vi "q-PCR report.vi"() -> ()   [LabVIEW 2017]
uses:
  <vilib>/addons/_office/excel.llb/Excel Get Data ([str]).vi
  <vilib>/Utility/NIReport.llb/Append Text Table to Report (wrap).vi
  <vilib>/Utility/NIReport.llb/NI_report.lvclass
  <vilib>/Utility/NIReport.llb/Excel/NI_Excel.lvclass
  <vilib>/addons/_office/NI_ReportGenerationToolkit.lvlib
panel:
  out "q-PCR Result":picture[][](array[picture])
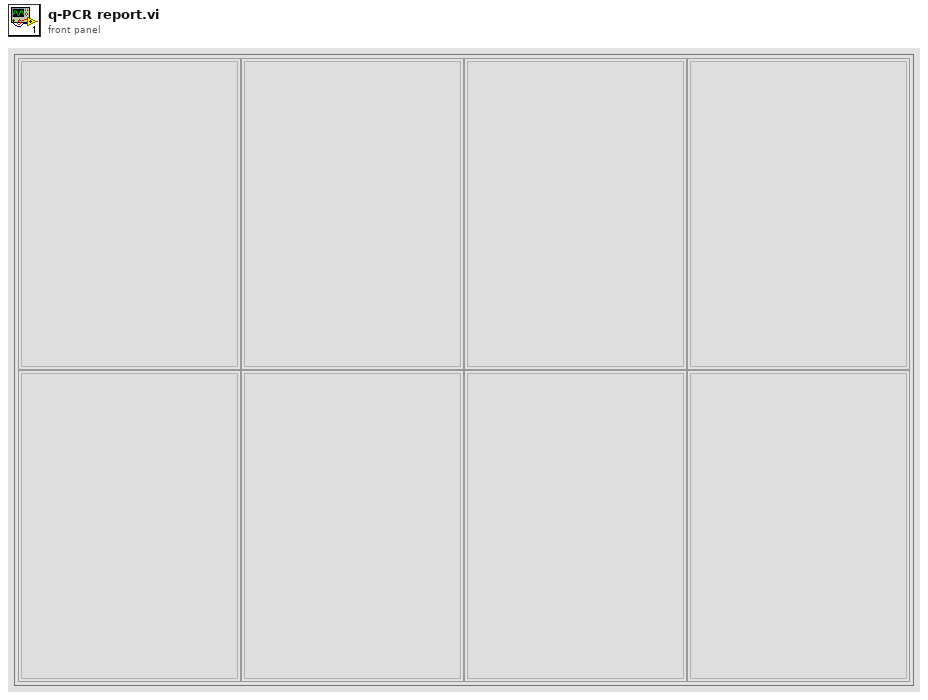
[diagram p1: front panel]
types:
  T1 = enum16{"Load File", "Plate Config", "Main Processing", "Report generation"}
  T2 = enum16{"maximized", "minimized", "normal", "no change"}
  T3 = enum16{"Standard Report", "HTML", "Word", "Excel"}
  T4 = cluster{"Group #":dbl, "Biological replicate":dbl, "Technical replicate":dbl}
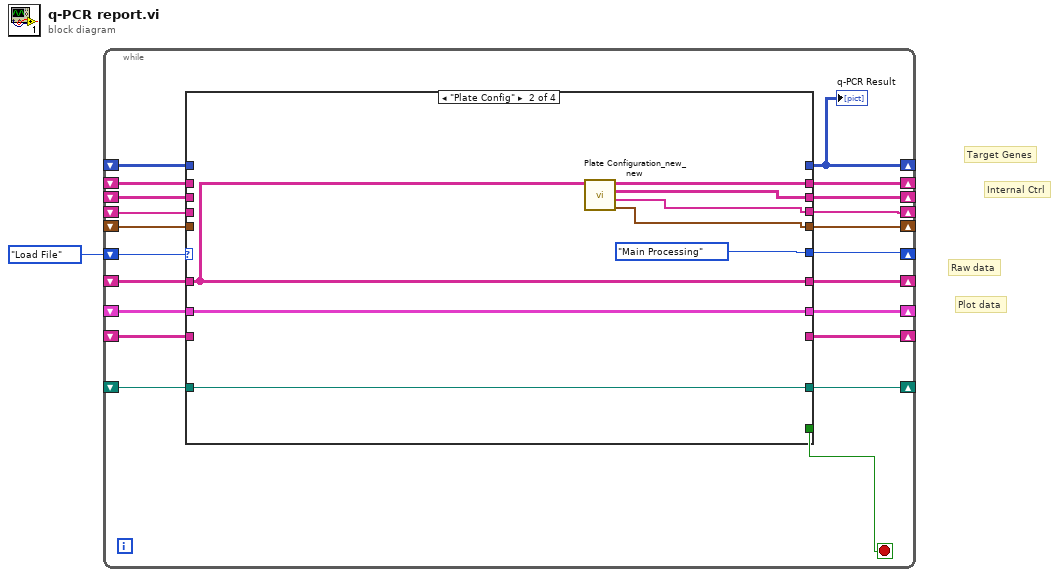
[diagram p0: block diagram]
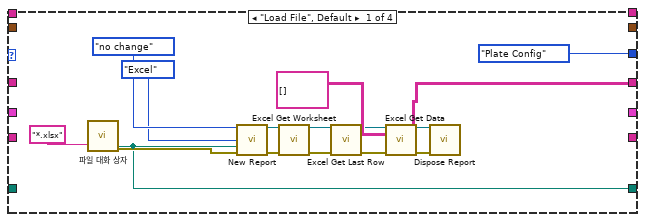
[diagram p2: hidden frame]
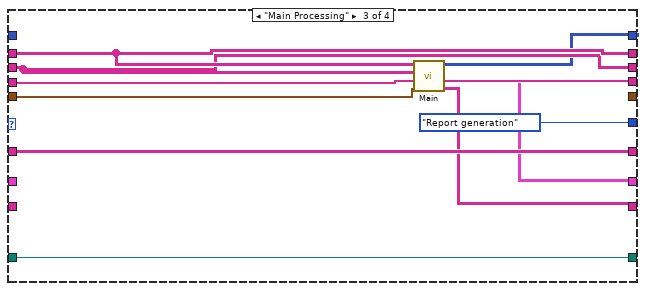
[diagram p3: hidden frame]
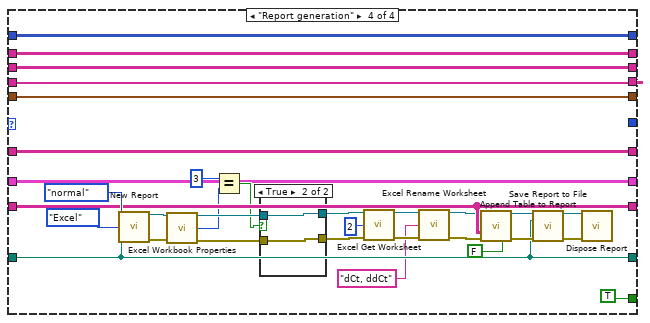
[diagram p4: hidden frame]
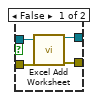
[diagram p5: hidden frame]
diagram:
  # "Plot data"
  # "Internal Ctrl"
  # "Target Genes"
  # "Raw data"
  n1 = while {
    shift-right: [w19] -> _
    shift-left: T1."Load File" -> [w22]
    shift-right: [w21] -> _
    shift-left: _ -> [w20]
    shift-right: [w18] -> _
    shift-left: _ -> [w14]
    shift-right: [w17] -> _
    shift-left: _ -> [w13]
    shift-right: [w16] -> _
    shift-left: _ -> [w12]
    shift-right: [w15] -> _
    shift-left: _ -> [w11]
    shift-right: [w8] -> _
    shift-left: _ -> [w9]
    shift-right: [w7] -> _
    shift-left: _ -> [w6]
    shift-right: [w5] -> _
    shift-left: _ -> [w4]
    shift-right: [w3] -> _
    shift-left: _ -> [w2]
    stop <- w10 stop-if-true
    n2 = case shown="\"Plate Config\"" w22 {
      tunnel: [w24 w45 w52 w83] -> w21
      tunnel: w20 -> [_ w45 w52 w83]
      tunnel: [T1."Plate Config" T1."Main Processing" T1."Report generation" _] -> w19
      tunnel: [_ w44 w55 w87] -> w18
      tunnel: [_ w43 w54 w86] -> w17
      tunnel: [_ w42 w53 w85] -> w16
      tunnel: [_ w41 _ w84] -> w15
      tunnel: w14 -> [_ _ w55 w87]
      tunnel: w13 -> [_ _ w54 w86]
      tunnel: w12 -> [_ _ w53 w85]
      tunnel: w11 -> [_ _ w56 w84]
      tunnel: [_ _ _ TRUE] -> w10
      tunnel: [_ _ w50 w82] -> w8
      tunnel: w9 -> [_ _ _ w82]
      tunnel: [w23 w40 w49 w72] -> w7
      tunnel: w6 -> [_ w40 w49 w72]
      tunnel: [_ _ w48 w76] -> w5
      tunnel: w4 -> [_ _ _ w76]
      tunnel: [_ w39 w47 w57] -> w3
      tunnel: w2 -> [_ w39 _ w57]
      frame "Load File", Default {
        w36 = "*.xlsx" ("pattern (all files)")
        n3 = call "파일 대화 상자"("pattern (all files)"=w36, "pattern label"=w36) -> ("selected path"=w23:path, "error out"=w35:errorcluster)  [unwired: 10 in, 2 out]
        n4 = call <vilib>:"New Report.vi"("window state (normal)"=T2."no change", "report type"=T3."Excel", "template (empty)"=w23, "error in (no error)"=w35) -> ("report out"=w26:refnum<class "NI_report.lvclass">, "error out"=w27:errorcluster)  [unwired: 10 in]
        n5 = call <vilib>:"Excel Get Worksheet.vi"("report in"=w26, "error in (no error)"=w27) -> ("report out"=w28:refnum<class "NI_report.lvclass">, "error out"=w34:errorcluster)  [unwired: 12 in]
        n6 = call <vilib>:"Excel Get Last Row.vi"("report in"=w28, "error in (no error)"=w34) -> ("report out"=w29:refnum<class "NI_report.lvclass">, "error out"=w33:errorcluster)  [unwired: 11 in, 1 out]
        n7 = call-poly <vilib>:"Excel Get Data.vi"("report in"=w29, "data type"=string[][] [], "error in (no error)"=w33) -> ("report out"=w31:refnum<class "NI_report.lvclass">, "data"=w24:string[][], "error out"=w32:errorcluster)  [unwired: 10 in]
        n8 = call-dynamic "Dispose Report.vi"("report in"=w31, "error in (no error)"=w32) -> ()  [unwired: 13 in, 1 out]
      }
      frame "Plate Config" {
        n9 = call "Plate Configuration_new_new.vi"("all rows"=w45) -> ("출력 클러스터"=w41:T4, "RowHdrs"=w42:string[], "Internal Ctrl"=w43:string[][], "Target Gene"=w44:string[][][])  [unwired: 3 in]
      }
      frame "Main Processing" {
        n10 = call "Main.vi"("출력 클러스터 2"=w56, "RowHdrs"=w53, "Internal Control"=w54, "Target Gene"=w55) -> ("Result"=w48:string[][], "Plot data"=w47:cluster{i32[], dbl[]}[][], "Bar (or symbol) plot"=w50:picture[][])  [unwired: 1 in]
      }
      frame "Report generation" {
        n11 = call <vilib>:"New Report.vi"("window state (normal)"=T2."normal", "report type"=T3."Excel", "template (empty)"=w72) -> ("report out"=w67:refnum<class "NI_report.lvclass">, "error out"=w69:errorcluster)  [unwired: 11 in]
        n12 = call <vilib>:"Excel Workbook Properties.vi"("report in"=w67, "error in (no error)"=w69) -> ("report out"=w66:refnum<class "NI_report.lvclass">, "worksheets count"=w65:i32, "error out"=w68:errorcluster)  [unwired: 10 in, 1 out]
        n13 = Equal?(x=3, y=w65) -> (x = y?=w63:bool)
        n14 = case shown="True" w63 {
          tunnel: [w92 w94] -> w79
          tunnel: [w91 w93] -> w78
          tunnel: w68 -> [w90 w93]
          tunnel: w66 -> [w89 w94]
          frame False {
            n15 = call <vilib>:"Excel Add Worksheet.vi"("report in"=w89, "error in (no error)"=w90) -> ("report out"=w92:refnum<class "NI_report.lvclass">, "error out"=w91:errorcluster)  [unwired: 12 in]
          }
          frame True {
          }
        }
        n16 = call <vilib>:"Excel Get Worksheet.vi"("report in"=w79, "worksheet index (0)"=2, "error in (no error)"=w78) -> ("report out"=w59:refnum<class "NI_report.lvclass">, "error out"=w62:errorcluster)  [unwired: 11 in]
        n17 = call <vilib>:"Excel Rename Worksheet.vi"("report in"=w59, "worksheet name (\"\")"="dCt, ddCt" ("worksheet name (\"\")"), "error in (no error)"=w62) -> ("report out"=w60:refnum<class "NI_report.lvclass">, "error out"=w61:errorcluster)  [unwired: 11 in]
        n18 = call-poly <vilib>:"Append Table to Report.vi"("report in"=w60, "text data"=w76, "error in (no error)"=w61, "show grid lines (YES)"=FALSE) -> ("report out"=w74:refnum<class "NI_report.lvclass">, "error out"=w73:errorcluster)  [unwired: 8 in, 2 out]
        n19 = call-dynamic "Save Report to File.vi"("report in"=w74, "report file path"=w72, "error in (no error)"=w73) -> ("report out"=w71:refnum<class "NI_report.lvclass">, "error out"=w70:errorcluster)  [unwired: 11 in]
        n20 = call-dynamic "Dispose Report.vi"("report in"=w71, "error in (no error)"=w70) -> ()  [unwired: 13 in, 1 out]
      }
    }
    "q-PCR Result" <- w8
  }
